vi "Send HTTP request.vi"(8 "error in (no error)":errorcluster, 11 "request":string) -> (0 "error out":errorcluster, 2 "headers":string, 3 "response":string)   [LabVIEW 2020, in "MCP Server tests.lvlib"]
uses:
  MCP Server tests.lvlib
  <vilib>/httpClient/POSTBuffer.vi
  <vilib>/httpClient/LabVIEWHTTPClient.lvlib
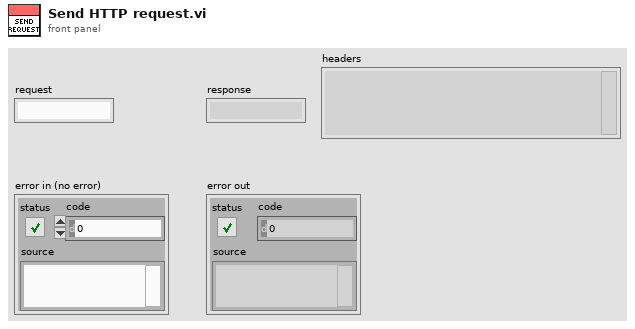
[diagram p1: front panel]
types:
  T1 = typedef "LabVIEWHTTPClient.lvlib/ClientHandle.ctl" = refnum<k1>
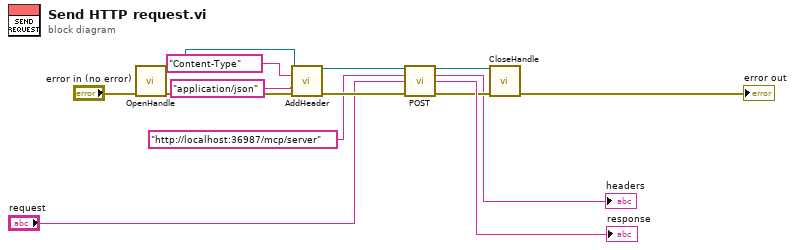
[diagram p0: block diagram]
diagram:
  n1 = call <vilib>:"OpenHandle.vi"("error in (no error)"="error in (no error)") -> ("client handle out"=w12:T1, "error out"=w11:errorcluster)  [unwired: 13 in]
  n2 = call <vilib>:"AddHeader.vi"("client handle"=w12, "header"="Content-Type", "value"="application/json", "error in (no error)"=w11) -> ("client handle out"=w9:T1, "error out"=w6:errorcluster)  [unwired: 10 in]
  n3 = call-poly <vilib>:"POST.vi"("client handle"=w9, "url"="http://localhost:36987/mcp/server", "buffer"="request", "error in (no error)"=w6) -> ("client handle out"=w14:T1, "headers"=→"headers":string, "body"=→"response":string, "error out"=w2:errorcluster)  [unwired: 8 in]
  n4 = call <vilib>:"CloseHandle.vi"("client handle"=w14, "error in (no error)"=w2) -> ("error out"=→"error out":errorcluster)  [unwired: 13 in]
